vi "Instrument Options.vi"(0 "VISA resource name":refnum<visa-resource-name>, 11 "error in (no error)":errorcluster) -> (4 "VISA resource name out":refnum<visa-resource-name>, 6 "Instrument Version":string, 10 "Options List":string, 15 "error out":errorcluster)   [LabVIEW 2020, in "Rohde&Schwarz RTx Oscilloscopes.lvlib"]
doc: "This VI returns the instrument version number and the list of options which the instrument is equipped with.\n\nRemote-control commands:\n*IDN?\n*OPT?"
uses:
  Rohde&Schwarz RTx Oscilloscopes.lvlib
  rsidr_core_global.vi
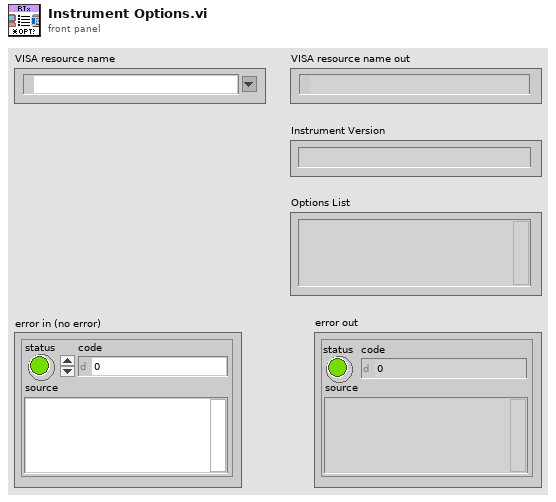
[diagram p1: front panel]
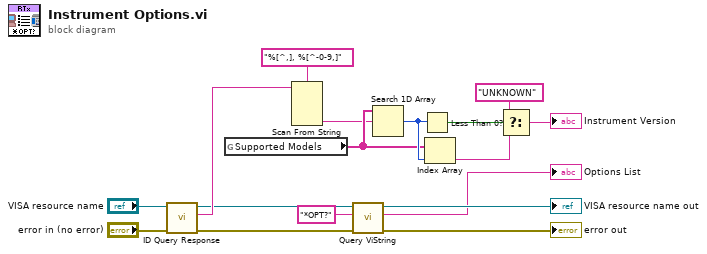
[diagram p0: block diagram]
diagram:
  n1 = call "ID Query Response.vi"("error in (no error)"="error in (no error)", "VISA resource name"="VISA resource name") -> ("error out"=w7:errorcluster, "ID Query Response"=w17:string, "VISA resource name out"=w3:refnum<visa-resource-name>)  [unwired: 7 in]
  n2 = global read "rsidr_core_global.vi" "Supported Models"() -> (w10:string[])
  n3 = Scan From String(format string="%[^,], %[^-0-9,]", input string=w17) -> (output 2=w2:string)  [unwired: 5 in, 3 out]
  n4 = call "Query ViString.vi"("error in (no error)"=w7, "Query"="*OPT?", "VISA resource name"=w3) -> ("error out"=→"error out":errorcluster, "Response Value"=→"Options List":string, "VISA resource name out"=→"VISA resource name out":refnum<visa-resource-name>)  [unwired: 6 in]
  n5 = Search 1D Array(1D array=w10, element=w2) -> (index of element=w11:i32)  [unwired: 1 in]
  n6 = Less Than 0?(x=w11) -> (x < 0?=w15:bool)
  n7 = Index Array(array=w10, index=w11) -> (element=w14:string)
  n8 = Select(t="UNKNOWN", s=w15, f=w14) -> (s? t:f=→"Instrument Version":string)
